vi "lastNSampWfms.vi"(6 "Time signal(s) in":waveform(dbl)[](array[waveform]), 8 "error in (no error)":errorcluster, 10 "Samples":u32, 11 "Instrument handle":refnum<k15>) -> (0 "error out":errorcluster, 3 "Instrument handle out":refnum<k15>, 4 "Shifted time signal(s)":waveform(dbl)[](array[waveform]))   [LabVIEW 2020]
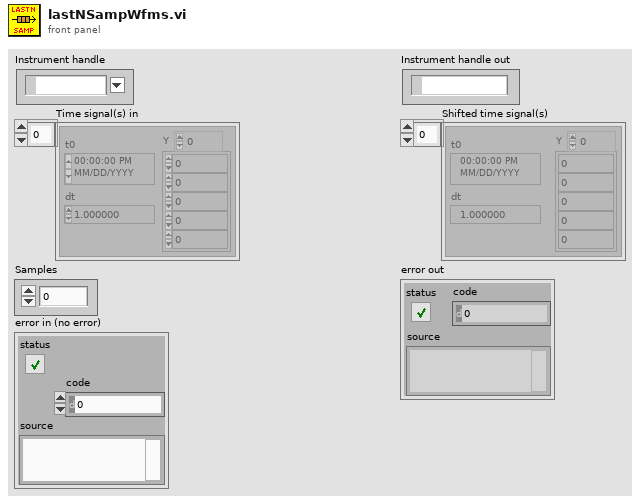
[diagram p1: front panel]
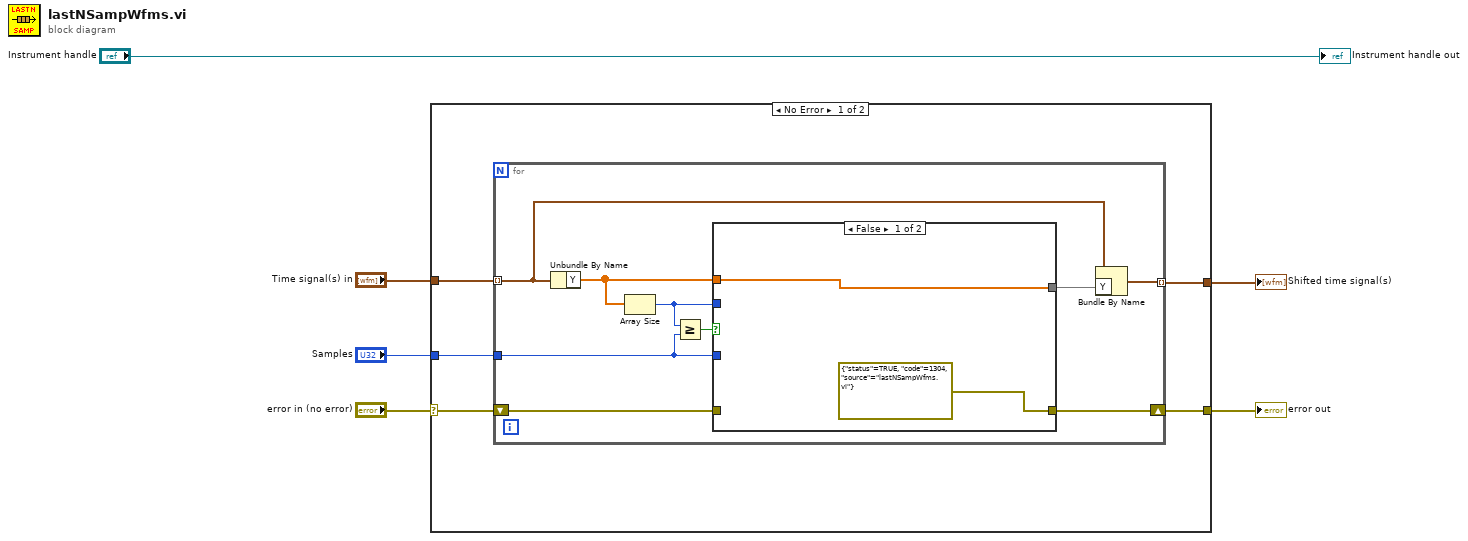
[diagram p0: block diagram]
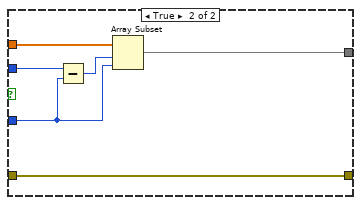
[diagram p2: hidden frame]
diagram:
  n1 = case shown="No Error" "error in (no error)" {
    selector: "error in (no error)" -> [w10 w30]
    tunnel: "Time signal(s) in" -> [w11 w29]
    tunnel: "Samples" -> [w9 _]
    tunnel: [w8 w30] -> w1
    tunnel: [w7 w29] -> w2
    frame No Error {
      n2 = for {
        tunnel: w11 -> [w12] mode=indexing
        shift-right: [w15] -> w8
        shift-left: w10 -> [w16]
        tunnel: w9 -> [w18]
        tunnel: [w13] -> w7 mode=indexing
        n3 = Unbundle By Name(w12) -> ("Y"=w20:dbl[])
        n4 = Array Size(array=w20) -> (size(s)=w17:i32)
        n5 = Greater Or Equal?(x=w17, y=w18) -> (x >= y?=w19:bool)
        n6 = case shown="False" w19 {
          tunnel: w17 -> [_ w28]
          tunnel: w20 -> [w22 w27]
          tunnel: w18 -> [_ w25]
          tunnel: w16 -> [_ w24]
          tunnel: [errorcluster {"status"=TRUE, "code"=1304, "source"="lastNSampWfms.vi"} ("error IO") w24] -> w15
          tunnel: [w22 w23] -> w14
          frame False {
          }
          frame True {
            n7 = Subtract(x=w28, y=w25) -> (x-y=w26:u32)
            n8 = Array Subset(array=w27, index=w26, length=w25) -> (w23:dbl[])
          }
        }
        n9 = Bundle By Name(cluster=w12, "Y"=w14) -> (w13:waveform(dbl))
      }
    }
    frame Error {
    }
  }
  "error out" <- w1
  "Shifted time signal(s)" <- w2
  "Instrument handle out" <- "Instrument handle"
